vi "c_Update adress ip.vi"() -> (1 "Case Label":T1)   [LabVIEW 2021, in "Maestro Control.lvclass"]
uses:
  Maestro Control.lvclass
  <vilib>/addons/_Workers/Library/Case Label.ctl
  <vilib>/addons/_Workers/Library/Workers.lvlib
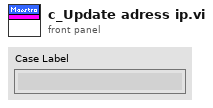
[diagram p1: front panel]
types:
  T1 = typedef "Workers.lvlib/Case Label.ctl" = string
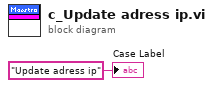
[diagram p0: block diagram]
diagram:
  "Case Label" <- T1 "Update adress ip" ("Case Label")
